vi "Store Channel Display.vi"(0 "Channels in":T1={"DAQ Settings"={"Trigger Type"=enum."Manual", "Trigger Samples"=0, "Pretrigger Samples"=0, "Trigger Interval"=0.0, "Time Units"=FALSE, "Auto Save"=FALSE, "Sample Rate"=7.0, "Select Analog"=FALSE, "Trigger Value"=0.0, "Trigger Stop Method"=enum."Use Samples Value to Stop Trigger", "Rate Sec/Min"=FALSE, "Save Mode"=enum."Single File", "File Size Limit"=0.0, "Log File Type"=enum."Basic", "Trigger Data Index"=0, "Log Rate"=7.0, "Rate Sec/Min (Log)"=FALSE, "Sample Rate (S/s)"=0.0, "Log Rate (S/s)"=0.0}, "Channels"=[], "Header"={"CA Number"="", "Test Name"="", "Serial Number"="", "Technician"=""}, "Graph Settings"={"Graph Labels"=[], [], [], [], [], [], [], [], [], [], [], [], [], "Graph Toggles"=[], "Axis Toggles"=[], "Graph Range"=enum."1"}, "Test Limits"=[], "All Type Info"=[], "Save Mode"=enum."Single File", "Data Base Path"=path ""} {"DAQ Settings"."Trigger Interval" min=0.0; "DAQ Settings"."Pretrigger Samples" min=0; "DAQ Settings"."Trigger Samples" min=0}, 5 "Channel Display":T11) -> (4 "Channels out":T1={"DAQ Settings"={"Trigger Type"=enum."Manual", "Trigger Samples"=0, "Pretrigger Samples"=0, "Trigger Interval"=0.0, "Time Units"=FALSE, "Auto Save"=FALSE, "Sample Rate"=7.0, "Select Analog"=FALSE, "Trigger Value"=0.0, "Trigger Stop Method"=enum."Use Samples Value to Stop Trigger", "Rate Sec/Min"=FALSE, "Save Mode"=enum."Single File", "File Size Limit"=0.0, "Log File Type"=enum."Basic", "Trigger Data Index"=0, "Log Rate"=7.0, "Rate Sec/Min (Log)"=FALSE, "Sample Rate (S/s)"=0.0, "Log Rate (S/s)"=0.0}, "Channels"=[], "Header"={"CA Number"="", "Test Name"="", "Serial Number"="", "Technician"=""}, "Graph Settings"={"Graph Labels"=[], [], [], [], [], [], [], [], [], [], [], [], [], "Graph Toggles"=[], "Axis Toggles"=[], "Graph Range"=enum."1"}, "Test Limits"=[], "All Type Info"=[], "Save Mode"=enum."Single File", "Data Base Path"=path ""} {"DAQ Settings"."Trigger Interval" min=0.0; "DAQ Settings"."Pretrigger Samples" min=0; "DAQ Settings"."Trigger Samples" min=0})   [LabVIEW 2023]
uses:
  Type Defs and Controls/Sensor List Cluster.ctl
  Type Defs and Controls/Channel Config Screen.ctl
  Type Defs and Controls/Sensor Config.ctl
  Type Defs and Controls/DAQ Settings.ctl
  Type Defs and Controls/Trigger Stop Method.ctl
  Type Defs and Controls/Log File Type.ctl
  Type Defs and Controls/Channel Config.ctl
  Type Defs and Controls/Header.ctl
  Type Defs and Controls/Graph Settings Type Def.ctl
  Type Defs and Controls/Test Limits.ctl
  Type Defs and Controls/All Part Info.ctl
  Type Defs and Controls/Part Info.ctl
panel:
  # "EGU"
  # "EGU"
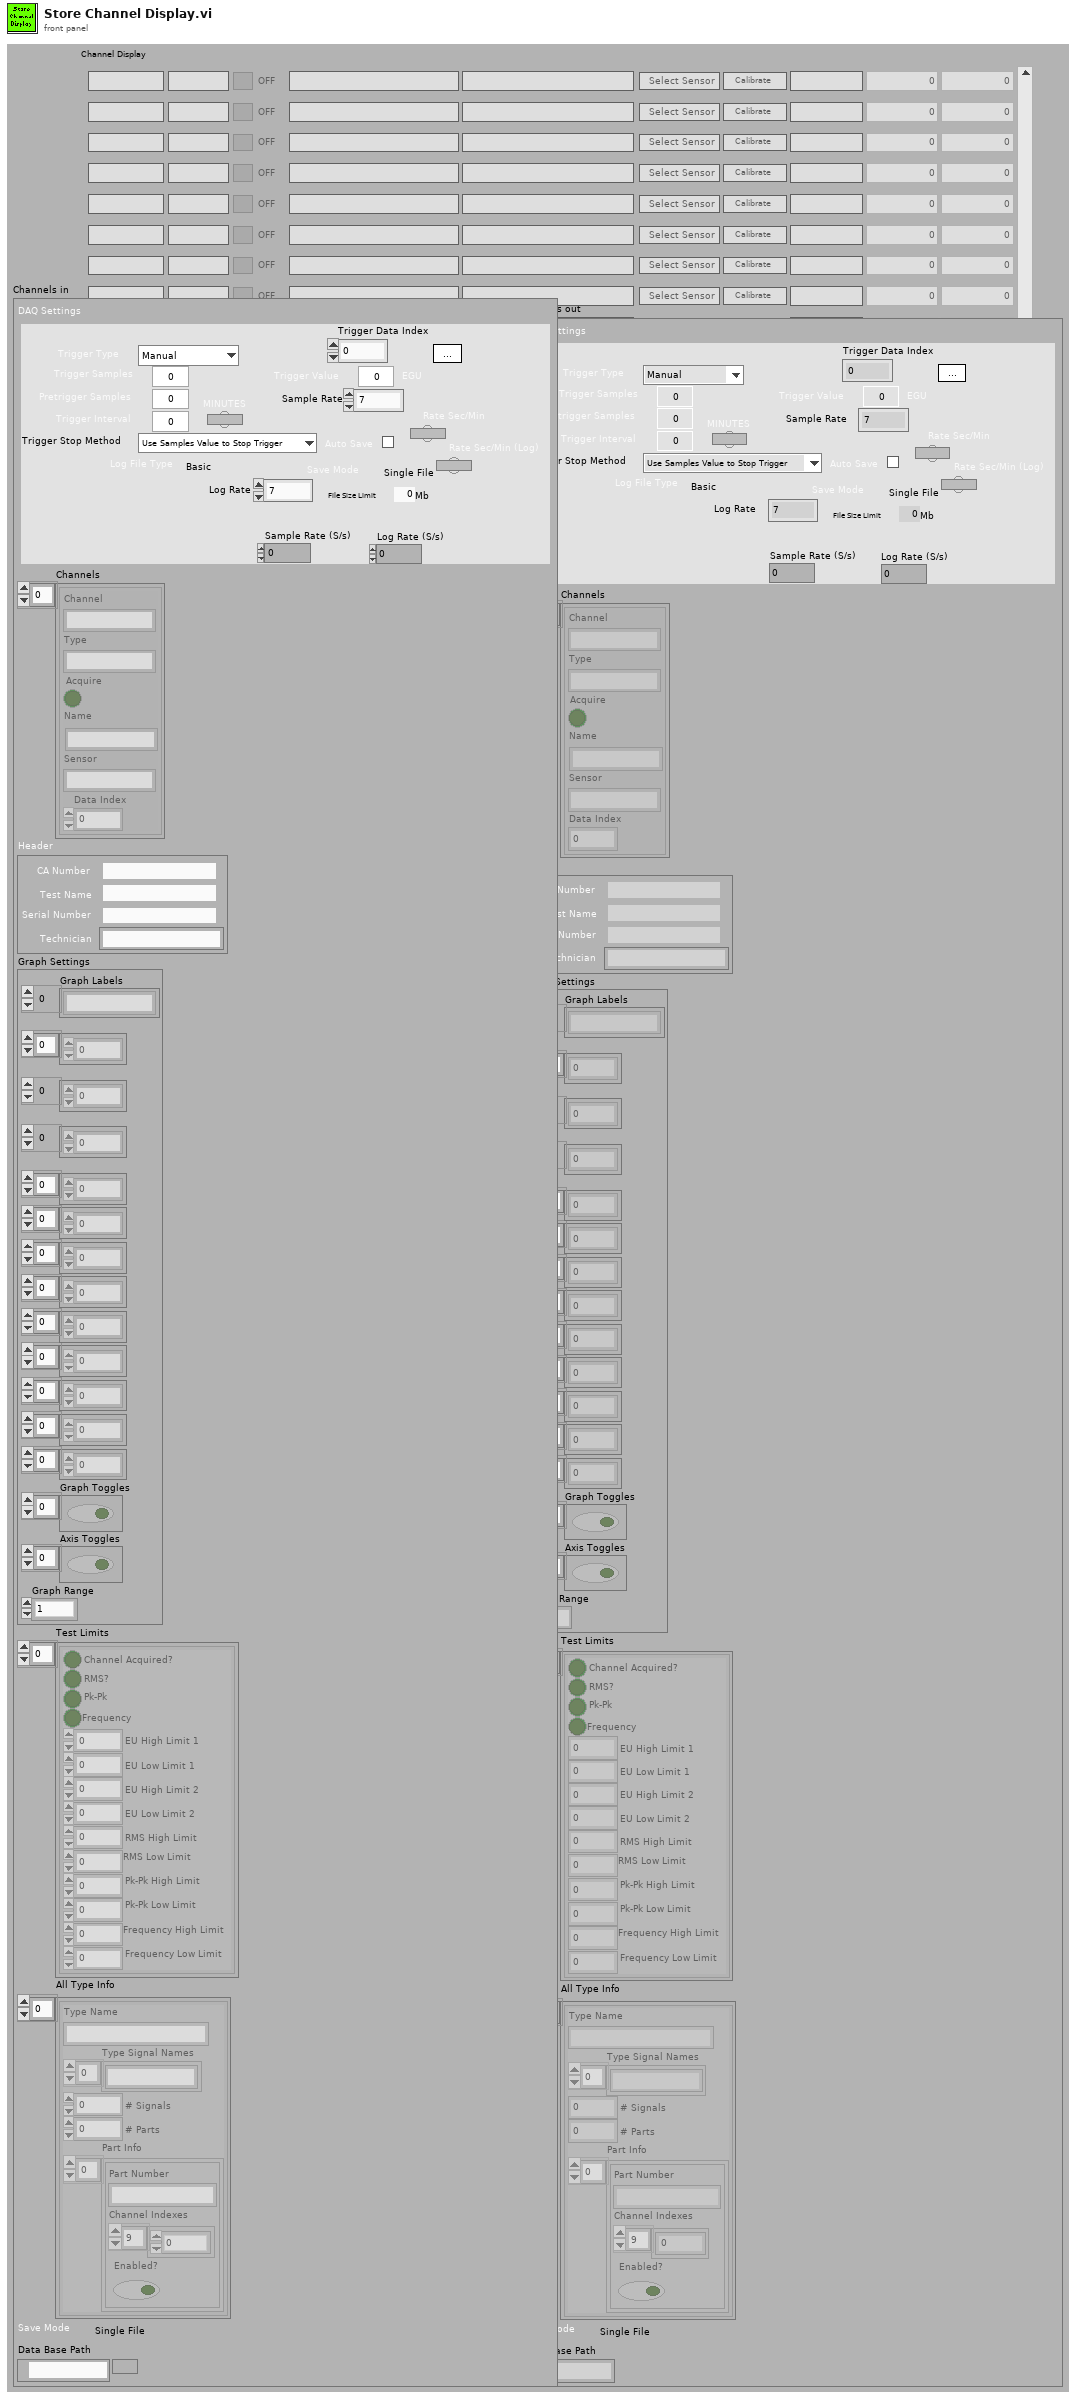
[diagram p1: front panel]
types:
  T1 = typedef "Sensor Config.ctl" = cluster{"DAQ Settings":T2, "Channels":T5[], "Header":T6, "Graph Settings":T7, "Test Limits":T8[], "All Type Info":T9, "Save Mode":enum16{"Single File", "Segmented Files", "New File at Midnight"}, "Data Base Path":path}
  T2 = typedef "DAQ Settings.ctl" = cluster{"Trigger Type":enum16{"Manual", "Timed", "Analog Rising", "Analog Falling"}, "Trigger Samples":i32, "Pretrigger Samples":i32, "Trigger Interval":dbl, "Time Units":bool, "Auto Save":bool, "Sample Rate":dbl, "Select Analog":bool, "Trigger Value":dbl, "Trigger Stop Method":T3, "Rate Sec/Min":bool, "Save Mode":enum16{"Single File", "Segmented Files", "New File at Midnight"}, "File Size Limit":dbl, "Log File Type":T4, "Trigger Data Index":u32, "Log Rate":dbl, "Rate Sec/Min (Log)":bool, "Sample Rate (S/s)":dbl, "Log Rate (S/s)":dbl}
  T3 = typedef "Trigger Stop Method.ctl" = enum16{"Use Samples Value to Stop Trigger", "Use Threshold to Stop Trigger"}
  T4 = typedef "Log File Type.ctl" = enum16{"Basic", "RTS"}
  T5 = typedef "Channel Config.ctl" = cluster{"Channel":string, "Type":string, "Acquire":bool, "Name":string, "Sensor":string, "Data Index":u32}
  T6 = typedef "Header.ctl" = cluster{"CA Number":string, "Test Name":string, "Serial Number":string, "Technician":string}
  T7 = typedef "Graph Settings Type Def.ctl" = cluster{"Graph Labels":string[], u8[], i16[], u32[], u8[], u8[], u8[], u32[], u8[], u8[], u8[], dbl[], dbl[], "Graph Toggles":bool[], "Axis Toggles":bool[], "Graph Range":enum16{"1", "2", "3", "4", "5", "10", "15", "30", "60"}}
  T8 = typedef "Test Limits.ctl" = cluster{"Channel Acquired?":bool, "RMS?":bool, "Pk-Pk":bool, "Frequency":bool, "EU High Limit 1":dbl, "EU Low Limit 1":dbl, "EU High Limit 2":dbl, "EU Low Limit 2":dbl, "RMS High Limit":dbl, "RMS Low Limit":dbl, "Pk-Pk High Limit ":dbl, "Pk-Pk Low Limit":dbl, "Frequency High Limit":dbl, "Frequency Low Limit":dbl}
  T9 = typedef "All Part Info.ctl" = cluster{"Type Name":string, "Type Signal Names":string[], "# Signals":i32, "# Parts":i32, "Part Info":T10[]}[]
  T10 = typedef "Part Info.ctl" = cluster{"Part Number":string, "Channel Indexes":u16[], "Enabled?":bool}
  T11 = typedef "Sensor List Cluster.ctl" = T12[]
  T12 = typedef "Channel Config Screen.ctl" = cluster{"Channel":string, "Description":string, "Acquire":bool, "Sensor":string, "Chg Sensor":bool, "Cal Date":string, "Offset":dbl, "Span":dbl, "Cal":bool, "Test Limits":bool, "Type":string, "Data Index":u32}
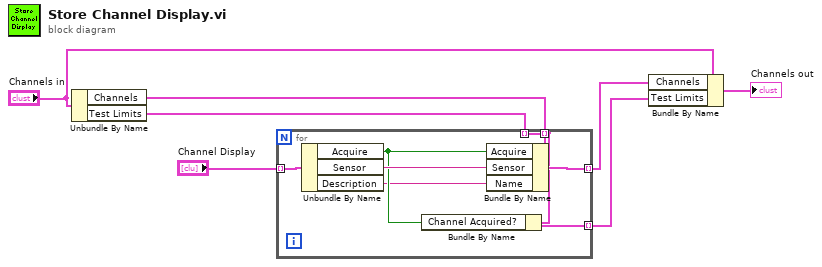
[diagram p0: block diagram]
diagram:
  n1 = Unbundle By Name("Channels in") -> ("Channels"=w4:T5[], "Test Limits"=w2:T8[])
  n2 = for {
    tunnel: "Channel Display" -> [w15] mode=indexing
    tunnel: [w14] -> w3 mode=indexing
    tunnel: w4 -> [w13] mode=indexing
    tunnel: [w11] -> _ mode=indexing
    tunnel: w2 -> [w11] mode=indexing
    tunnel: [w9] -> w1 mode=indexing
    n3 = Unbundle By Name(w15) -> ("Acquire"=w10:bool, "Sensor"=w12:string, "Description"=w8:string)
    n4 = Bundle By Name(cluster=w11, "Channel Acquired?"=w10) -> (w9:T8)
    n5 = Bundle By Name(cluster=w13, "Acquire"=w10, "Sensor"=w12, "Name"=w8) -> (w14:T5)
  }
  n6 = Bundle By Name(cluster="Channels in", "Channels"=w3, "Test Limits"=w1) -> (→"Channels out":T1)
